vi "CPU Temperature.vi"(8 "error in (no error)":errorcluster, 11 "RP Communicator in":refnum<class "RP Communicator.lvclass">) -> (0 "error out":errorcluster, 2 "CPU Temperature":dbl, 3 "RP Communicator out":refnum<class "RP Communicator.lvclass">)   [LabVIEW 2016, in "RP Communicator.lvclass"]
uses:
  RP Communicator.lvclass
  RP Communicator.lvclass/RP Communicator.ctl
  Read Timeout.vi
  RP Read Temperature TCP.vi
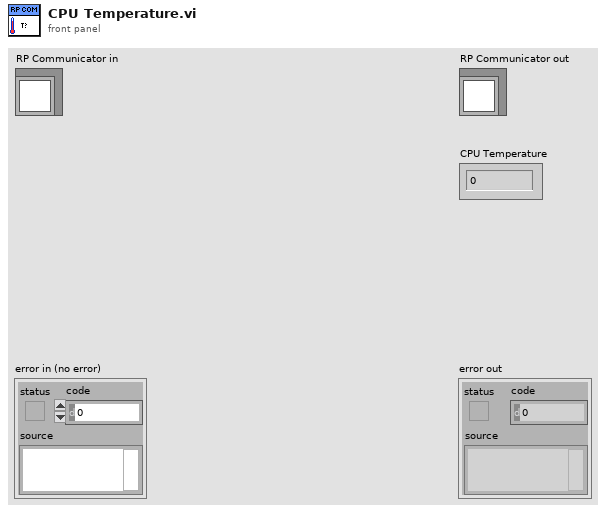
[diagram p1: front panel]
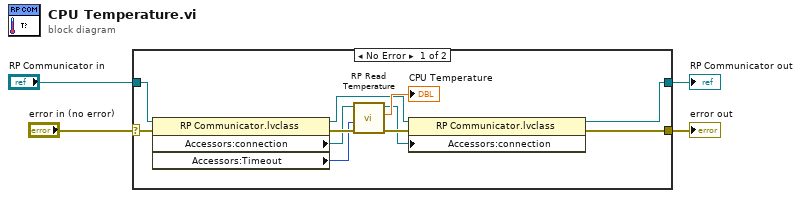
[diagram p0: block diagram]
diagram:
  n1 = case shown="No Error" "error in (no error)" {
    selector: "error in (no error)" -> [w15 w17]
    tunnel: [w8 w17] -> w3
    tunnel: [w7 w16] -> w1
    tunnel: "RP Communicator in" -> [w11 w16]
    frame No Error {
      n2 = property class="RP Communicator.lvclass"(reference=w11, error in=w15) -> (reference out=w10:refnum<class "RP Communicator.lvclass">, error out=w12:errorcluster, "Accessors:connection"=w9:refnum<k5>, "Accessors:Timeout"=w5:i32)
      n3 = call-poly "RP Read Temperature.vi"("Error In"=w12, "timeout ms (25000)"=w5, "connection ID"=w9) -> ("error out"=w14:errorcluster, "Thermometer"=→"CPU Temperature":dbl, "connection ID out"=w6:refnum<k5>)  [unwired: 6 in]
      n4 = property class="RP Communicator.lvclass"(reference=w10, error in=w14, "Accessors:connection"=w6) -> (reference out=w7:refnum<class "RP Communicator.lvclass">, error out=w8:errorcluster)
    }
    frame Error {
    }
  }
  "error out" <- w3
  "RP Communicator out" <- w1
